vi "products.vi"(3 "speed in":i32(listbox), 4 "PACKAGE TYPE in":T2, 5 "Cluster in":T1) -> (1 "Cluster out":T1)   [LabVIEW 2026]
uses:
  packagingytpee.ctl
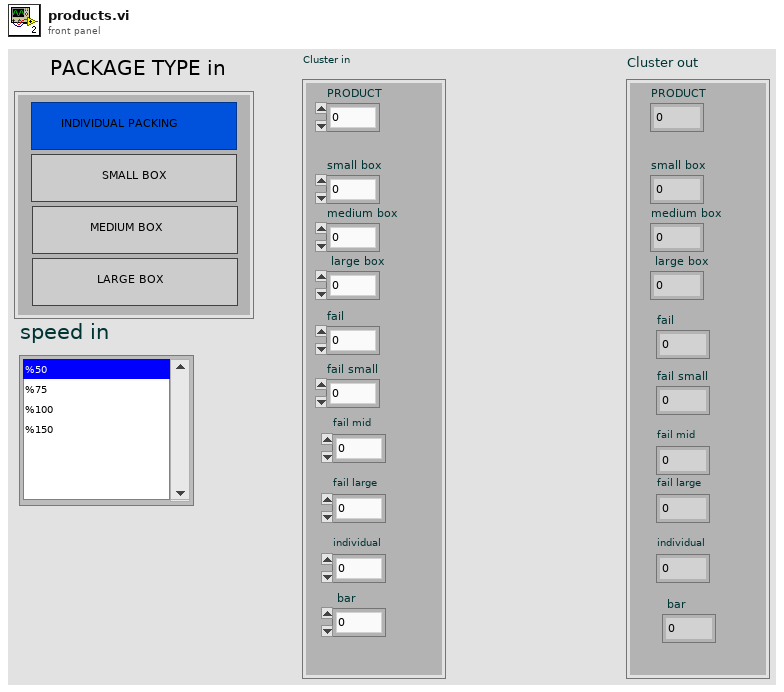
[diagram p1: front panel]
types:
  T1 = cluster{"PRODUCT":u16, "small box":u16, "medium box":u16, " large box":u16, "fail":u16, "fail small":u16, "fail mid":u16, "fail large":u16, "individual":u16, " bar ":u8}
  T2 = typedef "packagingytpee.ctl" = enum32{"İNDİVİDUAL", "SMALL", "MID", "LARGE"}
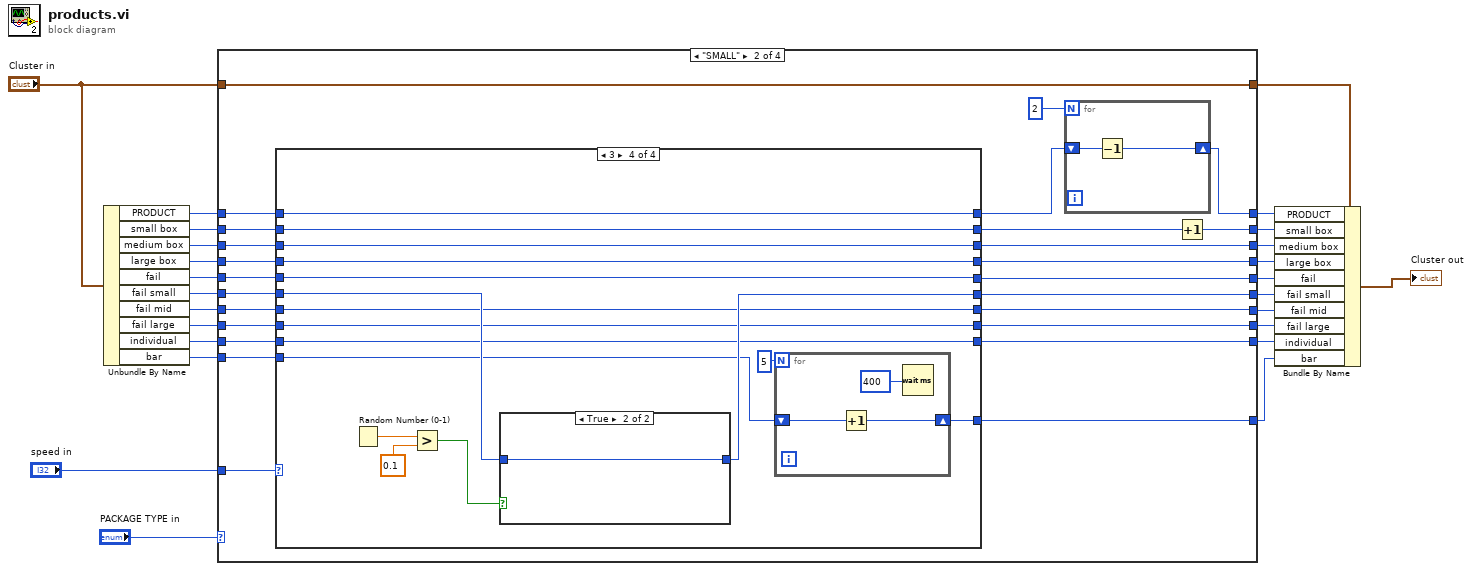
[diagram p0: block diagram]
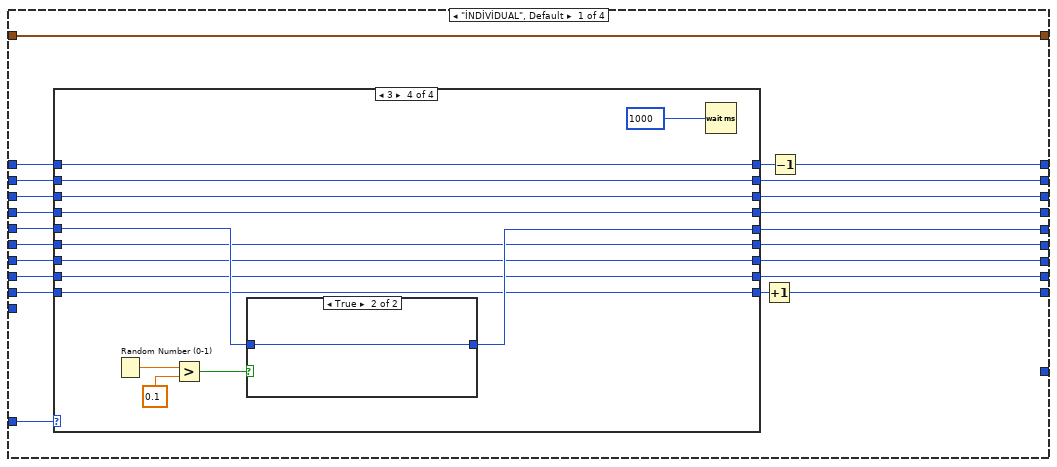
[diagram p2: hidden frame]
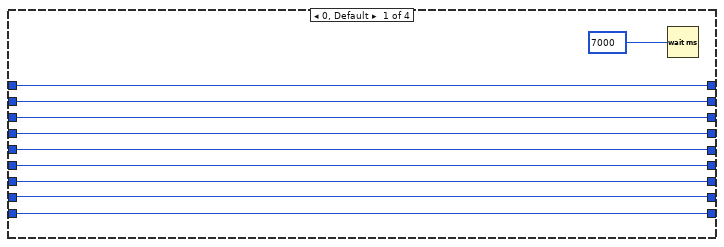
[diagram p3: hidden frame]
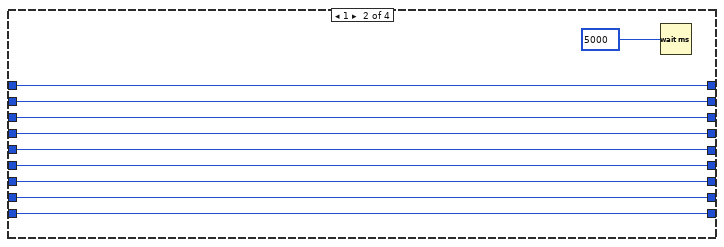
[diagram p4: hidden frame]
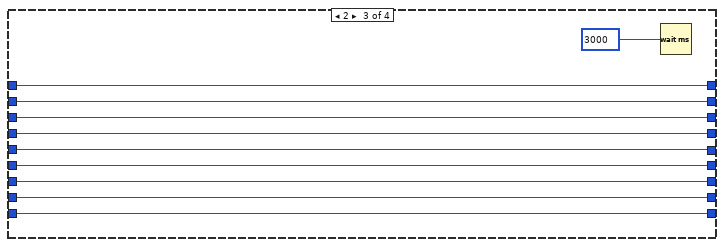
[diagram p5: hidden frame]
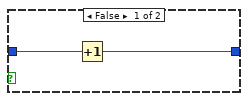
[diagram p6: hidden frame]
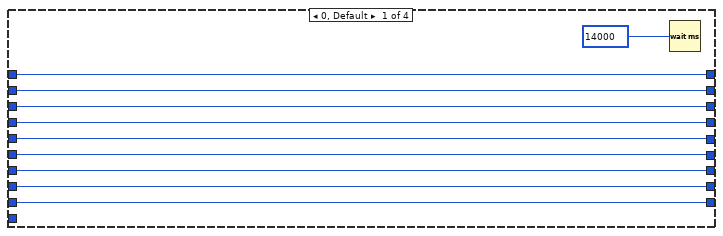
[diagram p7: hidden frame]
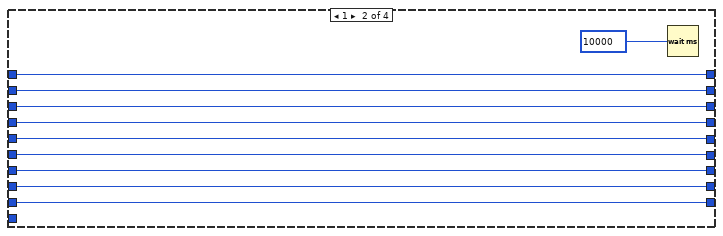
[diagram p8: hidden frame]
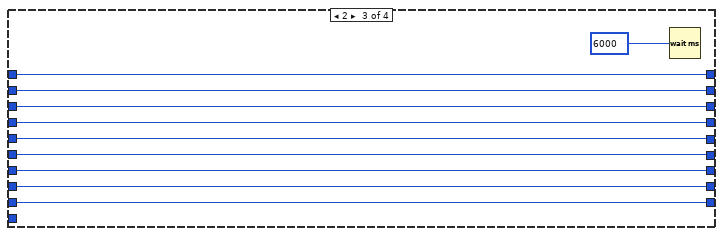
[diagram p9: hidden frame]
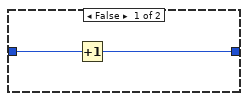
[diagram p10: hidden frame]
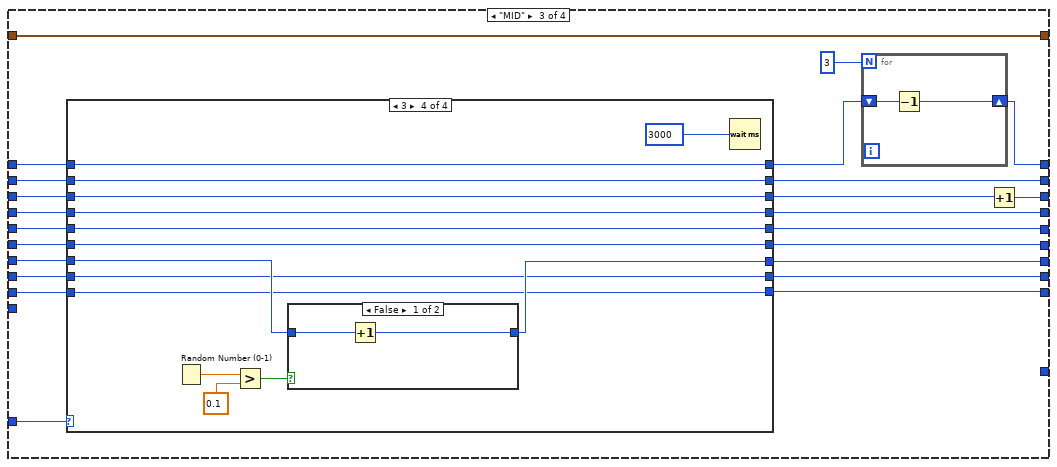
[diagram p11: hidden frame]
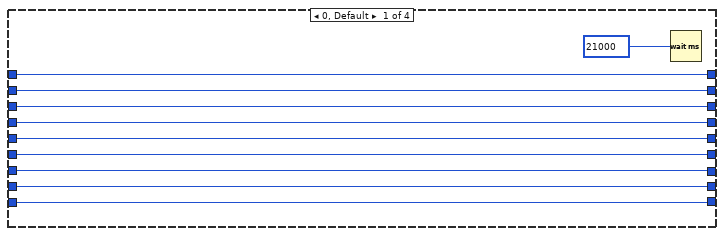
[diagram p12: hidden frame]
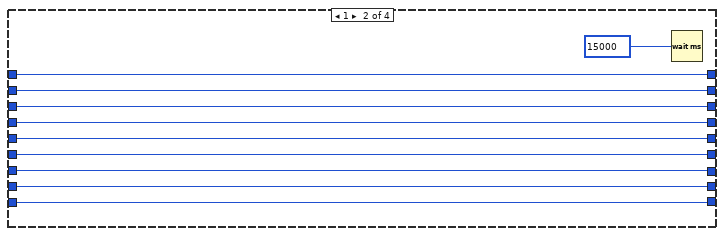
[diagram p13: hidden frame]
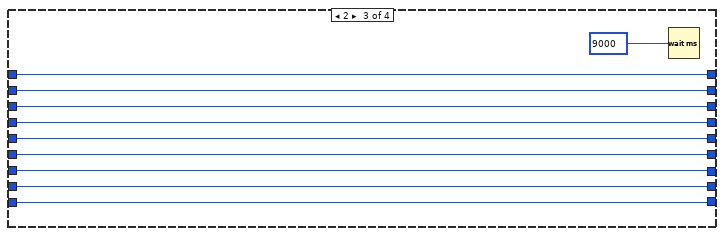
[diagram p14: hidden frame]
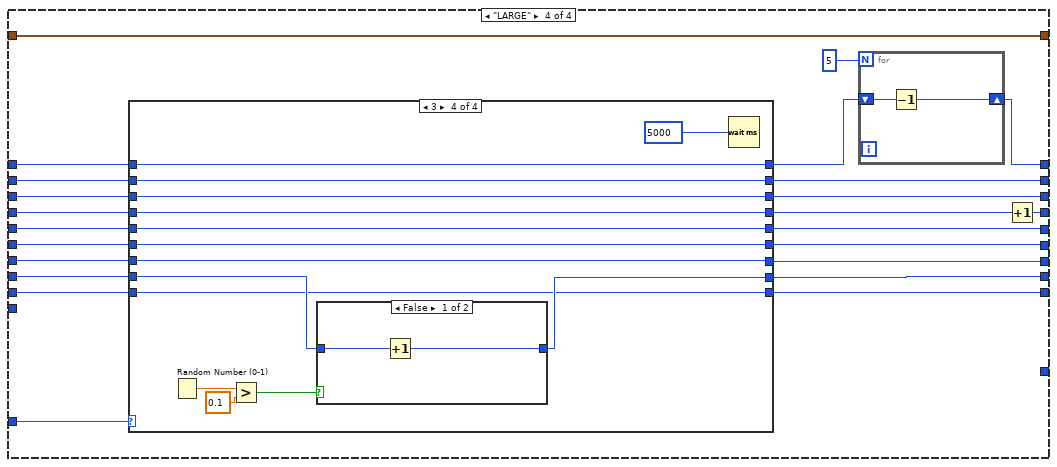
[diagram p16: hidden frame]
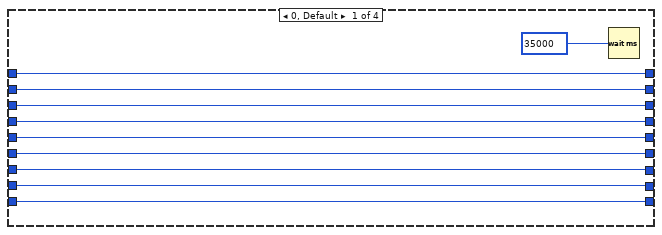
[diagram p17: hidden frame]
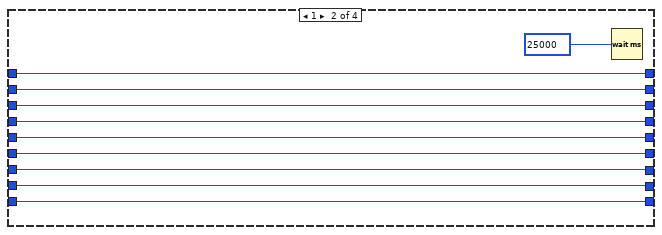
[diagram p18: hidden frame]
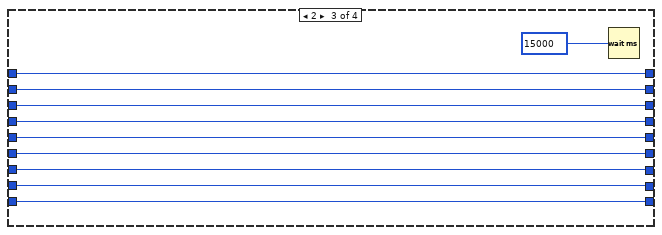
[diagram p19: hidden frame]
diagram:
  n1 = Unbundle By Name("Cluster in") -> ("PRODUCT"=w25:u16, "small box"=w22:u16, "medium box"=w21:u16, "large box"=w20:u16, "fail"=w12:u16, "fail small"=w10:u16, "fail mid"=w8:u16, "fail large"=w6:u16, "individual"=w4:u16, "bar"=w2:u8)
  n2 = case shown="\"SMALL\"" "PACKAGE TYPE in" {
    tunnel: "Cluster in" -> [w37 w115 w192 w264]
    tunnel: w25 -> [w46 w119 w196 w268]
    tunnel: [w37 w115 w192 w264] -> w13
    tunnel: "speed in" -> [w47 w107 w186 w259]
    tunnel: w22 -> [w44 w118 w195 w267]
    tunnel: w21 -> [w43 w117 w194 w266]
    tunnel: w20 -> [w42 w116 w193 w265]
    tunnel: [w41 w110 w188 w261] -> w19
    tunnel: [w40 w108 w187 w260] -> w18
    tunnel: [w39 w114 w184 w258] -> w17
    tunnel: [w38 w113 w191 w257] -> w16
    tunnel: w12 -> [w36 w106 w183 w255]
    tunnel: [w35 w105 w182 w254] -> w11
    tunnel: w10 -> [w34 w104 w181 w253]
    tunnel: [w33 w103 w180 w252] -> w9
    tunnel: w8 -> [w32 w102 w179 w251]
    tunnel: [w31 w101 w178 w250] -> w7
    tunnel: w6 -> [w30 w100 w177 w249]
    tunnel: [w29 w99 w176 w248] -> w5
    tunnel: w4 -> [w28 w98 w175 w247]
    tunnel: [w26 w97 w174 w246] -> w3
    tunnel: w2 -> [_ w96 _ _]
    tunnel: [_ w95 _ _] -> w1
    frame "İNDİVİDUAL", Default {
      n3 = case shown="3" w47 {
        tunnel: w46 -> [w56 w66 w76 w90]
        tunnel: [w56 w66 w76 w90] -> w45
        tunnel: w44 -> [w55 w65 w75 w89]
        tunnel: [w55 w65 w75 w89] -> w40
        tunnel: w43 -> [w54 w64 w74 w88]
        tunnel: [w54 w64 w74 w88] -> w39
        tunnel: w42 -> [w53 w63 w73 w87]
        tunnel: [w53 w63 w73 w87] -> w38
        tunnel: w36 -> [w52 w62 w72 w83]
        tunnel: [w52 w62 w72 w82] -> w35
        tunnel: w34 -> [w51 w61 w71 w81]
        tunnel: [w51 w61 w71 w81] -> w33
        tunnel: [w50 w60 w70 w80] -> w31
        tunnel: w32 -> [w50 w60 w70 w80]
        tunnel: w30 -> [w49 w59 w69 w79]
        tunnel: [w49 w59 w69 w79] -> w29
        tunnel: [w48 w58 w68 w78] -> w27
        tunnel: w28 -> [w48 w58 w68 w78]
        frame 0, Default {
          n4 = Wait (ms)(milliseconds to wait=u32 7000) -> ()  [unwired: 1 out]
        }
        frame 1 {
          n5 = Wait (ms)(milliseconds to wait=u32 5000) -> ()  [unwired: 1 out]
        }
        frame 2 {
          n6 = Wait (ms)(milliseconds to wait=u32 3000) -> ()  [unwired: 1 out]
        }
        frame 3 {
          n7 = Random Number (0-1)() -> (number: 0 to 1=w86:dbl)
          n8 = Greater?(x=w86, y=0.1) -> (0:w84:bool)
          n9 = case shown="True" w84 {
            tunnel: w83 -> [w93 w94]
            tunnel: [w92 w94] -> w82
            frame False {
              n10 = Increment(x=w93) -> (x+1=w92:u16)
            }
            frame True {
            }
          }
          n11 = Wait (ms)(milliseconds to wait=u32 1000) -> ()  [unwired: 1 out]
        }
      }
      n12 = Increment(x=w27) -> (x+1=w26:u16)
      n13 = Decrement(x=w45) -> (x-1=w41:u16)
    }
    frame "SMALL" {
      n14 = case shown="3" w107 {
        tunnel: w119 -> [w127 w137 w147 w164]
        tunnel: w118 -> [w128 w140 w150 w167]
        tunnel: [w128 w140 w150 w167] -> w109
        tunnel: w117 -> [w130 w139 w149 w166]
        tunnel: [w130 w139 w149 w166] -> w114
        tunnel: w116 -> [w129 w138 w148 w165]
        tunnel: [w129 w138 w148 w165] -> w113
        tunnel: [w127 w137 w147 w164] -> w111
        tunnel: w106 -> [w126 w136 w146 w163]
        tunnel: [w126 w136 w146 w163] -> w105
        tunnel: w104 -> [w125 w135 w145 w159]
        tunnel: [w125 w135 w145 w158] -> w103
        tunnel: w102 -> [w124 w134 w144 w157]
        tunnel: [w124 w134 w144 w157] -> w101
        tunnel: [w123 w133 w143 w156] -> w99
        tunnel: w100 -> [w123 w133 w143 w156]
        tunnel: [w122 w132 w142 w155] -> w97
        tunnel: w98 -> [w122 w132 w142 w155]
        tunnel: w96 -> [_ _ _ w153]
        tunnel: [_ _ _ w152] -> w95
        frame 0, Default {
          n15 = Wait (ms)(milliseconds to wait=u32 14000) -> ()  [unwired: 1 out]
        }
        frame 1 {
          n16 = Wait (ms)(milliseconds to wait=u32 10000) -> ()  [unwired: 1 out]
        }
        frame 2 {
          n17 = Wait (ms)(milliseconds to wait=u32 6000) -> ()  [unwired: 1 out]
        }
        frame 3 {
          n18 = Random Number (0-1)() -> (number: 0 to 1=w162:dbl)
          n19 = Greater?(x=w162, y=0.1) -> (0:w160:bool)
          n20 = case shown="True" w160 {
            tunnel: w159 -> [w172 w173]
            tunnel: [w171 w173] -> w158
            frame False {
              n21 = Increment(x=w172) -> (x+1=w171:u16)
            }
            frame True {
            }
          }
          n22 = for {
            N: 5 -> [_]
            shift-right: [w168] -> w152
            shift-left: w153 -> [w169]
            n23 = Increment(x=w169) -> (x+1=w168:u8)
            n24 = Wait (ms)(milliseconds to wait=u32 400) -> ()  [unwired: 1 out]
          }
        }
      }
      n25 = for {
        N: 2 -> [_]
        shift-right: [w120] -> w110
        shift-left: w111 -> [w121]
        n26 = Decrement(x=w121) -> (x-1=w120:u16)
      }
      n27 = Increment(x=w109) -> (x+1=w108:u16)
    }
    frame "MID" {
      n28 = case shown="3" w186 {
        tunnel: w196 -> [w204 w214 w224 w238]
        tunnel: w195 -> [w205 w217 w227 w241]
        tunnel: [w205 w217 w227 w241] -> w187
        tunnel: w194 -> [w207 w216 w226 w240]
        tunnel: [w207 w216 w226 w240] -> w185
        tunnel: w193 -> [w206 w215 w225 w239]
        tunnel: [w206 w215 w225 w239] -> w191
        tunnel: [w204 w214 w224 w238] -> w189
        tunnel: w183 -> [w203 w213 w223 w237]
        tunnel: [w203 w213 w223 w237] -> w182
        tunnel: w181 -> [w202 w212 w222 w236]
        tunnel: [w202 w212 w222 w236] -> w180
        tunnel: w179 -> [w201 w211 w221 w232]
        tunnel: [w201 w211 w221 w231] -> w178
        tunnel: w177 -> [w200 w210 w220 w230]
        tunnel: [w200 w210 w220 w230] -> w176
        tunnel: [w199 w209 w219 w229] -> w174
        tunnel: w175 -> [w199 w209 w219 w229]
        frame 0, Default {
          n29 = Wait (ms)(milliseconds to wait=u32 21000) -> ()  [unwired: 1 out]
        }
        frame 1 {
          n30 = Wait (ms)(milliseconds to wait=u32 15000) -> ()  [unwired: 1 out]
        }
        frame 2 {
          n31 = Wait (ms)(milliseconds to wait=u32 9000) -> ()  [unwired: 1 out]
        }
        frame 3 {
          n32 = Random Number (0-1)() -> (number: 0 to 1=w235:dbl)
          n33 = Greater?(x=w235, y=0.1) -> (0:w233:bool)
          n34 = case shown="False" w233 {
            tunnel: w232 -> [w244 w245]
            tunnel: [w243 w245] -> w231
            frame False {
              n35 = Increment(x=w244) -> (x+1=w243:u16)
            }
            frame True {
            }
          }
          n36 = Wait (ms)(milliseconds to wait=u32 3000) -> ()  [unwired: 1 out]
        }
      }
      n37 = for {
        N: 3 -> [_]
        shift-right: [w197] -> w188
        shift-left: w189 -> [w198]
        n38 = Decrement(x=w198) -> (x-1=w197:u16)
      }
      n39 = Increment(x=w185) -> (x+1=w184:u16)
    }
    frame "LARGE" {
      n40 = case shown="3" w259 {
        tunnel: w268 -> [w276 w286 w296 w310]
        tunnel: w267 -> [w277 w289 w299 w313]
        tunnel: [w277 w289 w299 w313] -> w260
        tunnel: w266 -> [w279 w288 w298 w312]
        tunnel: [w279 w288 w298 w312] -> w258
        tunnel: w265 -> [w278 w287 w297 w311]
        tunnel: [w278 w287 w297 w311] -> w256
        tunnel: [w276 w286 w296 w310] -> w262
        tunnel: w255 -> [w275 w285 w295 w309]
        tunnel: [w275 w285 w295 w309] -> w254
        tunnel: w253 -> [w274 w284 w294 w308]
        tunnel: [w274 w284 w294 w308] -> w252
        tunnel: [w273 w283 w293 w307] -> w250
        tunnel: w251 -> [w273 w283 w293 w307]
        tunnel: w249 -> [w272 w282 w292 w303]
        tunnel: [w272 w282 w292 w302] -> w248
        tunnel: [w271 w281 w291 w301] -> w246
        tunnel: w247 -> [w271 w281 w291 w301]
        frame 0, Default {
          n41 = Wait (ms)(milliseconds to wait=u32 35000) -> ()  [unwired: 1 out]
        }
        frame 1 {
          n42 = Wait (ms)(milliseconds to wait=u32 25000) -> ()  [unwired: 1 out]
        }
        frame 2 {
          n43 = Wait (ms)(milliseconds to wait=u32 15000) -> ()  [unwired: 1 out]
        }
        frame 3 {
          n44 = Random Number (0-1)() -> (number: 0 to 1=w306:dbl)
          n45 = Greater?(x=w306, y=0.1) -> (0:w305:bool)
          n46 = case shown="False" w305 {
            tunnel: w303 -> [w316 w317]
            tunnel: [w315 w317] -> w302
            frame False {
              n47 = Increment(x=w316) -> (x+1=w315:u16)
            }
            frame True {
            }
          }
          n48 = Wait (ms)(milliseconds to wait=u32 5000) -> ()  [unwired: 1 out]
        }
      }
      n49 = for {
        N: 5 -> [_]
        shift-right: [w269] -> w261
        shift-left: w262 -> [w270]
        n50 = Decrement(x=w270) -> (x-1=w269:u16)
      }
      n51 = Increment(x=w256) -> (x+1=w257:u16)
    }
  }
  n52 = Bundle By Name(cluster=w13, "PRODUCT"=w19, "small box"=w18, "medium box"=w17, "large box"=w16, "fail"=w11, "fail small"=w9, "fail mid"=w7, "fail large"=w5, "individual"=w3, "bar"=w1) -> (→"Cluster out":T1)
